vi "DPC_Plot_Data.vi"(4 "error in":errorcluster, 5 "Sreg_In":u16[][](array[numeric]), 6 "DataIn":u16[][](array[numeric]), 7 "tdms file in":refnum<k34>) -> (0 "error out":errorcluster, 1 "Sreg_Out":u16[][](array[numeric]), 3 "tdms file out":refnum<k34>)   [LabVIEW 2019]
uses:
  SiPM_Tests_Global_Var.vi
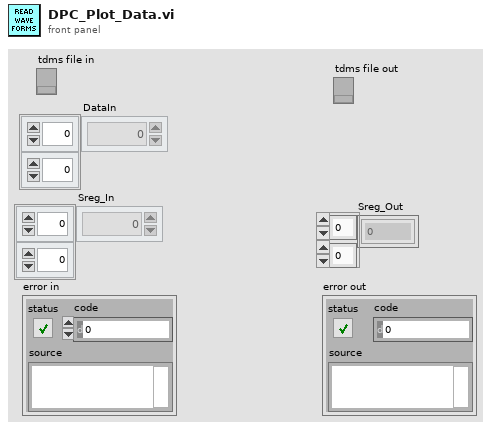
[diagram p1: front panel]
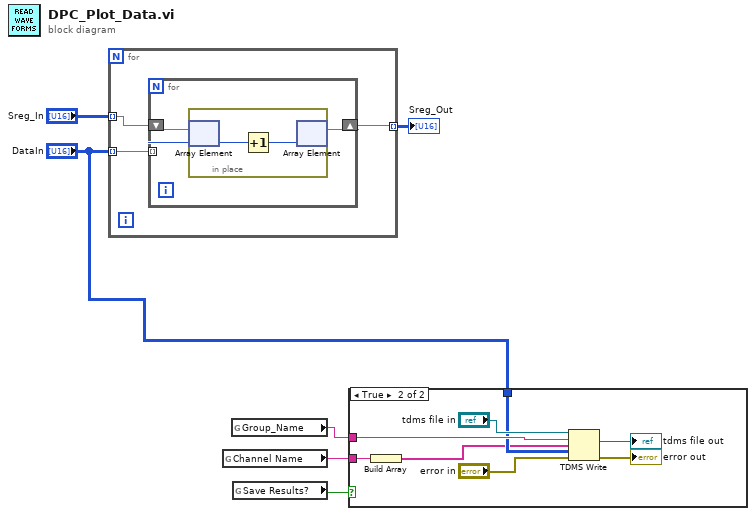
[diagram p0: block diagram]
diagram:
  n1 = for {
    tunnel: "DataIn" -> [w9] mode=indexing
    tunnel: "Sreg_In" -> [w8] mode=indexing
    tunnel: [w7] -> w2 mode=indexing
    n2 = for {
      tunnel: w9 -> [w12] mode=indexing
      shift-right: [w10] -> w7
      shift-left: w8 -> [w11]
      n3 = in-place {
        n4 = in-place-array #1(w11, w12) -> (w14:u16)
        n5 = Increment(x=w14) -> (x+1=w13:u16)
        n6 = in-place-array #1(w13) -> (w10:u16[])  [unwired: 1 out]
      }
    }
  }
  "Sreg_Out" <- w2
  n7 = global read "SiPM_Tests_Global_Var.vi" "Channel Name"() -> (w4:string)
  n8 = global read "SiPM_Tests_Global_Var.vi" "Group_Name"() -> (w5:string)
  n9 = global read "SiPM_Tests_Global_Var.vi" "Save Results?"() -> (w6:bool)
  n10 = case shown="True" w6 {
    tunnel: "DataIn" -> [_ w16]
    tunnel: w5 -> [_ w18]
    tunnel: w4 -> [_ w17]
    frame False {
    }
    frame True {
      n11 = Build Array(w17) -> (w15:string[])
      n12 = TDMS Write(0:"tdms file in", 5:w18, 7:w15, 9:w16, 11:"error in") -> (4:→"tdms file out":refnum<k34>, 15:→"error out":errorcluster)  [unwired: 1 in, 2 out]
    }
  }
